vi "get command from counter cluster.vi"(6 "tracking?":bool, 7 "counting photons?":bool, 10 "counter cluster":T2) -> (2 "command":T1)   [LabVIEW 2010]
uses:
  counter_cluster_tagResonant.ctl
  scan message.ctl
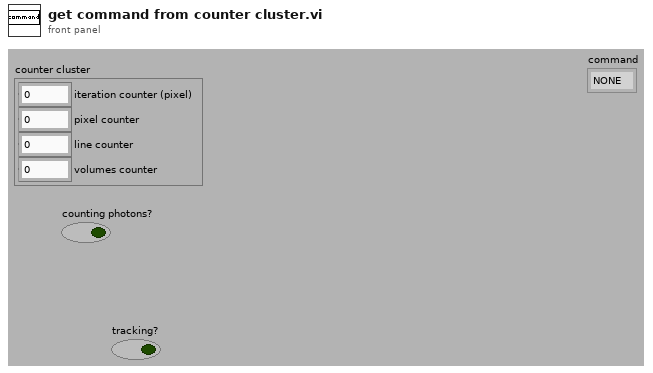
[diagram p1: front panel]
types:
  T1 = typedef "scan message.ctl" = enum8{"NONE", "VOLUME START", "LINE START", "XKALMAN", "YKALMAN", "ZKALMAN", "LINE START TRACKING"}
  T2 = typedef "counter_cluster_tagResonant.ctl" = cluster{"iteration counter (pixel)":u16, "pixel counter":u16, "line counter":i16, "volumes counter":u16}
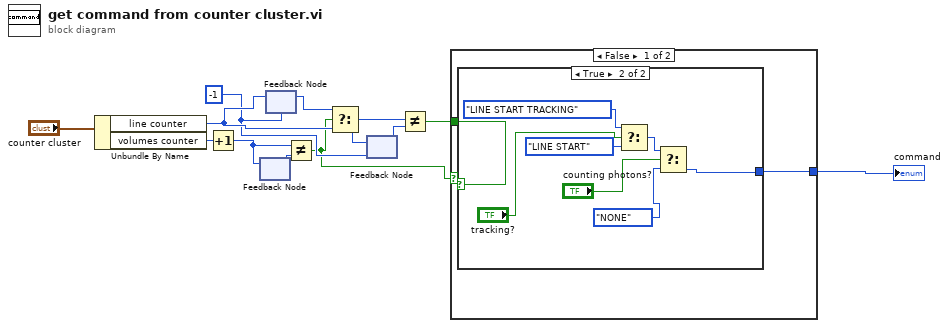
[diagram p0: block diagram]
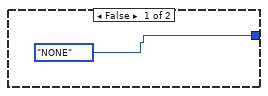
[diagram p2: hidden frame]
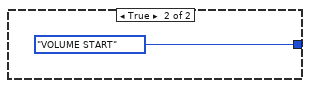
[diagram p3: hidden frame]
diagram:
  w4 = i16 -1 ("line counter")
  n1 = Unbundle By Name("counter cluster") -> ("line counter"=w8:i16, "volumes counter"=w10:u16)
  n2 = Increment(x=w10) -> (x+1=w1:u16)
  n3 = feedback #1() -> (w9:u16)  [unwired: 1 in]
  n4 = feedback-in #1(w1) -> ()
  n5 = feedback #2(w4) -> (w7:i16)
  n6 = feedback-in #2(w8) -> ()
  n7 = Not Equal?(x=w1, y=w9) -> (x != y?=w3:bool)
  n8 = Select(t=w7, s=w3, f=w8) -> (s? t:f=w5:i16)
  n9 = feedback #3(w4) -> (w6:i16)
  n10 = feedback-in #3(w5) -> ()
  n11 = Not Equal?(x=w5, y=w6) -> (x != y?=w2:bool)
  n12 = case shown="False" w3 {
    tunnel: [w13 scan_message."VOLUME START" ("Enum")] -> w11
    tunnel: w2 -> [w14 _]
    frame False {
      n13 = case shown="True" w14 {
        tunnel: [scan_message."NONE" ("f") w22] -> w13
        frame False {
        }
        frame True {
          n14 = Select(t=scan_message."LINE START TRACKING" ("Enum"), s="tracking?", f=scan_message."LINE START" ("Enum")) -> (s? t:f=w17:T1)
          n15 = Select(t=w17, s="counting photons?", f=scan_message."NONE") -> (s? t:f=w22:T1)
        }
      }
    }
    frame True {
    }
  }
  "command" <- w11
